vi "ADC Offset Gain_original.vi"(8 "error in (no error)":errorcluster, 9 "Sequence parameters":string[][](array[string])=[["Min limit", "Max limit", "Register sheet file", "Register Sheet"], ["", "", "CC2600.xls", "TX_BLE;Trim"], ["Reg write (addr;value)", "Operating frequency [Hz]", "", ""], ["NA", "2.44G", "", ""]], 10 "Run type":i32, 11 "Method parameters":T3={"Dev"={"Do not disturb DUT"=FALSE, "XOSC"=32000000.0, "Board type"="", "EM"="", "Configure tempboard"=TRUE, "Device specific info"=[], "Generic Object"=refnum}, "Method"={"Run type"=1, "Test name"="Current LPM2 4", "Comment"="", "Results folder"="", "AFC"=enum."Off", "Method name"="Current LPM2 4", "Method results"={"Excel brief report"=FALSE, "Spotfire report"=FALSE, "Starfish report"=FALSE}, "Operator"="", "Reference time"=timestamp(0 s since 1904-01-01), "AFC delay"=0.0, "Initialization"=enum."Enabled", "MD5 Sum"="", "HW addon board"=enum."None", "AFC Regsheet"="", "AFC Regfile"=path "", "dummy"=0.0}, "Inst"={"Instr"={"PS1"={"Name"="", "GPIB address"="", "VISA session"=""}, "PS2"={"Name"="", "GPIB address"="", "VISA session"=""}, "TC1"={"Name"="", "GPIB address"="", "VISA session"=""}, "TC2"={"Name"="", "GPIB address"="", "VISA session"=""}, "SA1"={"Name"="", "GPIB address"="", "VISA session"=""}, "SA2"={"Name"="", "GPIB address"="", "VISA session"=""}, "SG1"={"Name"="", "GPIB address"="", "VISA session"=""}, "SG2"={"Name"="", "GPIB address"="", "VISA session"=""}, "SG3"={"Name"="", "GPIB address"="", "VISA session"=""}, "MI1"={"Name"="", "GPIB address"="", "VISA session"=""}, "MI2"={"Name"="", "GPIB address"="", "VISA session"=""}, "SW SA"={"Name"="", "Controller addr"=""}, "SW SG"={"Name"="", "Controller addr"=""}, "MI3"={"Name"="", "GPIB address"="", "VISA session"=""}}, "Switchbox"={"RF Path"=0, "Cal compensation"=enum."TX", "Switchbox gain mode"="", "State"=enum."TX"}, "Instr to control (i.e. SA1)"="Default", "Intrument info string"=""}, "Sequence parameters"=[["Weight", "Min Limit", "Max Limit", "Register Sheet", "", "", "", "", "", "", "", "", ""], ["Vital", "", "1", "LPM2", "", "", "", "", "", "", "", "", ""], ["Resolution", "Reg write (addr;value)", "Chip mode", "Range", "", "", "", "", "", "", "", "", ""], ["u", "NA", "", "auto", "", "", "", "", "", "", "", "", ""]], "Cond"={"Temp logged"=25.0, "VDD1_PS1_6V"=-999.0, "VDD2_PS1_25V"=-999.0, "VDD4_PS2_25V"=-999.0, "VDD3_PS2_6V"=-999.0}, "Meas config"={"X-axis inner loop index"=32000000, "Y-axis outer loop index"=32000000, "X-axis"=[], "Y-axis"=[], "X-axis array req size"=32000000, "Y-axis array req size"=32000000, "Param description"=[], "Use meas clust for reporting"=FALSE, "Parameter index (page)"=0, "X-axis name"="", "Y-axis name"=""}} {"Cond"."VDD3_PS2_6V" format="%.3f"; "Cond"."VDD4_PS2_25V" format="%.3f"; "Cond"."VDD2_PS1_25V" format="%.3f"; "Cond"."VDD1_PS1_6V" format="%.3f"; "Method"."dummy" format="%.1p"; "Method"."AFC delay" format="%.1p"; "Dev"."XOSC" format="%.3p"}) -> (0 "error out":errorcluster, 1 "End method error":T2, 2 "Short Results":string[](array[string])=["0.00", "0.00", "0.00", "0.00"], 3 "Result summary":string[][](array[string])=[["Critical", "Output Power@2405 MHz", "-3", "4", "dBm"], ["Critical", "Output Power@2410 MHz", "-3", "4", "dBm"]])   [LabVIEW 2019]
doc: "[AutoDocStart]Performs crystal accuracy measurements. Measures the offset from ideal frequency. Primarily used for tuning XOSC capacitors and verifying XOSC trims.\n\nSweeping parameters: operating frequency, OSC override value and VDDR level\n\nResults: Offset frequency in ppm[AutoDocEnd]"
uses:
  User Lib/Utilities/Cluster definitions/Method input.ctl
  User Lib/Utilities/Cluster definitions/Device specific info.ctl
  User Lib/Utilities/Controls/Automatic Frequency Compensation types.ctl
  User Lib/Utilities/Controls/Method Reports.ctl
  User Lib/Utilities/Cluster definitions/Method Initialization.ctl
  User Lib/Utilities/Controls/HW addon boards.ctl
  User Lib/Utilities/Cluster definitions/Instr clust.ctl
  User Lib/Utilities/Switchbox control/SwitchBox_State._ENUMctl.ctl
  User Lib/Utilities/Cluster definitions/End method error cluster.ctl
  User Lib/Utilities/Cluster definitions/DUT vdd control.ctl
  User Lib/Utilities/Cluster definitions/DUT VDD4.ctl
  User Lib/Utilities/Cluster definitions/DUT VDD3.ctl
  User Lib/Utilities/Cluster definitions/DUT VDD2.ctl
  User Lib/Utilities/Cluster definitions/DUT VDD1.ctl
  User Lib/Generic chip methods/Classes/Generic_EM/Chameleon/Loki/Loki.lvclass
  5dbb33b4-abf2-4dec-afba-afc32014483e.vi
  7ebe6cd1-31d9-46d5-9500-a426c9f4248b.vi
  <vilib>/Utility/error.llb/Clear Errors.vi
  User Lib/Generic chip methods/Classes/Generic_EM/Chameleon/65nm.lvclass
  C:/Kharon/User Lib/Generic chip methods/Classes/Generic_EM/Generic_EM/Generic_EM.lvclass
  User Lib/Generic chip methods/board_to_chip_type.vi
  User Lib/Generic chip methods/Classes/Get_Class_init.vi
  User Lib/Generic chip methods/Classes/Generic_EM/Generic_EM/Generic_EM.lvclass
  <vilib>/Analysis/NI_AALPro.lvlib
panel:
  out "Max":u32
  out "Min":u32
  in  "Tab Control":T1(tab)
  out "Output Response [All DUTs]":u32[][](array[numeric])
  out "Measure Codes":dbl[](array[numeric])
  out "intercept":dbl
  out "slope":dbl
  out "Offset Error (mV)":dbl
  out "Gain Error (LSB)":dbl
  # "°C"
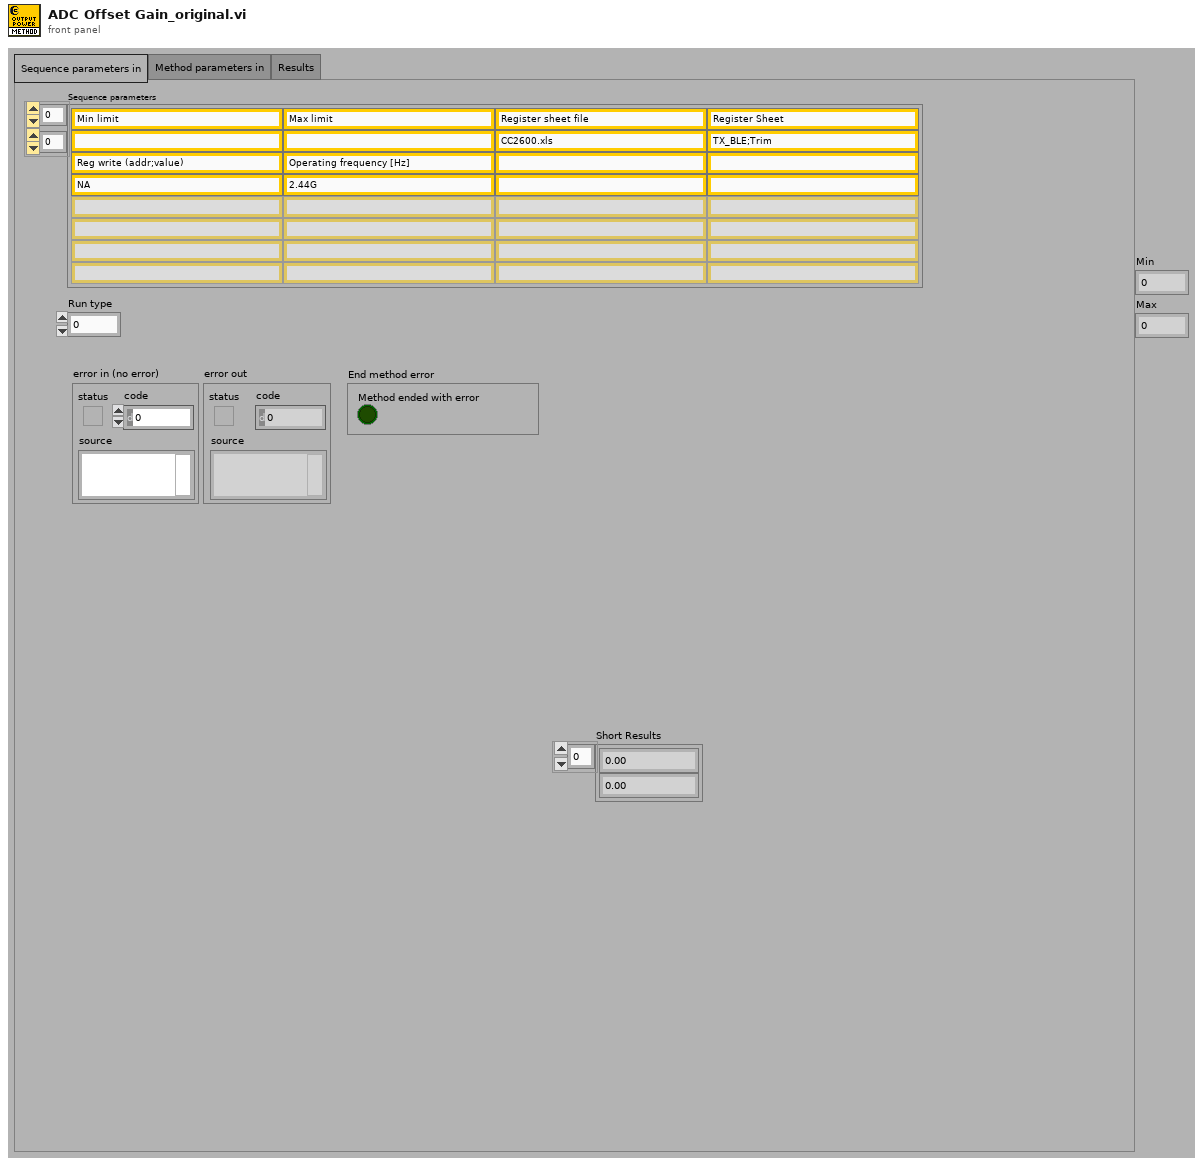
[diagram p1: front panel]
types:
  T1 = enum32{"Sequence parameters in", "Method parameters in", "Results"}
  T2 = typedef "End method error cluster.ctl" = cluster{"Method ended with error":bool}
  T3 = typedef "Method input.ctl" = cluster{"Dev":cluster{"Do not disturb DUT":bool, "XOSC":dbl, "Board type":string, "EM":string, "Configure tempboard":bool, "Device specific info":T4[], "Generic Object":refnum<class>}, "Method":cluster{"Run type":i32, "Test name":string, "Comment":string, "Results folder":string, "AFC":T5, "Method name":string, "Method results":T6, "Operator":string, "Reference time":timestamp, "AFC delay":dbl, "Initialization":T7, "MD5 Sum":string, "HW addon board":T8, "AFC Regsheet":string, "AFC Regfile":path, "dummy":dbl}, "Inst":T9, "Sequence parameters":string[][], "Cond":cluster{"Temp logged":dbl, "VDD1_PS1_6V":dbl, "VDD2_PS1_25V":dbl, "VDD4_PS2_25V":dbl, "VDD3_PS2_6V":dbl}, "Meas config":cluster{"X-axis inner loop index":i32, "Y-axis outer loop index":i32, "X-axis":string[], "Y-axis":string[], "X-axis array req size":i32, "Y-axis array req size":i32, "Param description":string[][], "Use meas clust for reporting":bool, "Parameter index (page)":i32, "X-axis name":string, "Y-axis name":string}}
  T4 = typedef "Device specific info.ctl" = cluster{"EM number":u8, "IP address":string, "Enabled":bool, "Slot no":u8, "RF path":u8, "EM name":string, "Wafer info":string, "AFC frequency ppm":dbl, "Register writes":string[][], "Meas data":string[][][], "Device comment":string}
  T5 = typedef "Automatic Frequency Compensation types.ctl" = enum16{"Off", "Compensate Instrument frequency", "Compensate DUT frequency", "Predictive - Compensate Instrument frequency", "Predictive - Compensate DUT frequency", "Do not skip re-init - Compensate Instrument frequency", "Do not skip re-init - Compensate DUT frequency"}
  T6 = typedef "Method Reports.ctl" = cluster{"Excel brief report":bool, "Spotfire report":bool, "Starfish report":bool}
  T7 = typedef "Method Initialization.ctl" = enum16{"Enabled", "Skip Instr and Device Init", "Enabled with Separate Flash", "Set PS, Device Init and Skip Instr Init", "Skip Device Init"}
  T8 = typedef "HW addon boards.ctl" = enum16{"None", "Current meas 5EM", "Stresstest 10EM"}
  T9 = typedef "Instr clust.ctl" = cluster{"Instr":cluster{"PS1":cluster{"Name":string, "GPIB address":string, "VISA session":refnum<visa-resource-name>}, "PS2":cluster{"Name":string, "GPIB address":string, "VISA session":refnum<visa-resource-name>}, "TC1":cluster{"Name":string, "GPIB address":string, "VISA session":refnum<visa-resource-name>}, "TC2":cluster{"Name":string, "GPIB address":string, "VISA session":refnum<visa-resource-name>}, "SA1":cluster{"Name":string, "GPIB address":string, "VISA session":refnum<visa-resource-name>}, "SA2":cluster{"Name":string, "GPIB address":string, "VISA session":refnum<visa-resource-name>}, "SG1":cluster{"Name":string, "GPIB address":string, "VISA session":refnum<visa-resource-name>}, "SG2":cluster{"Name":string, "GPIB address":string, "VISA session":refnum<visa-resource-name>}, "SG3":cluster{"Name":string, "GPIB address":string, "VISA session":refnum<visa-resource-name>}, "MI1":cluster{"Name":string, "GPIB address":string, "VISA session":refnum<visa-resource-name>}, "MI2":cluster{"Name":string, "GPIB address":string, "VISA session":refnum<visa-resource-name>}, "SW SA":cluster{"Name":string, "Controller addr":string}, "SW SG":cluster{"Name":string, "Controller addr":string}, "MI3":cluster{"Name":string, "GPIB address":string, "VISA session":refnum<visa-resource-name>}}, "Switchbox":cluster{"RF Path":i32, "Cal compensation":enum16{"TX", "RX", "Interferer", "No compensation", "Interferer2"}, "Switchbox gain mode":string, "State":T10}, "Instr to control (i.e. SA1)":string, "Intrument info string":string}
  T10 = typedef "SwitchBox_State._ENUMctl.ctl" = enum16{"TX", "RX", "SP:TX", "SP:RX", "SW:TX", "SW:RX"}
  T11 = typedef "DUT vdd control.ctl" = cluster{"VDD4 config":T12, "VDD3 config":T13, "VDD2 config":T14, "VDD1 config":T15}
  T12 = typedef "DUT VDD4.ctl" = u16
  T13 = typedef "DUT VDD3.ctl" = u16
  T14 = typedef "DUT VDD2.ctl" = u16
  T15 = typedef "DUT VDD1.ctl" = u16
  T16 = typedef "TFW ResponseData.ctl" = cluster{"errorCode":u32, "executionTime":u32, "processedCmdWord":u32, "responsePar":u32[], "actionCode":u32, "cmdStatus":u16}
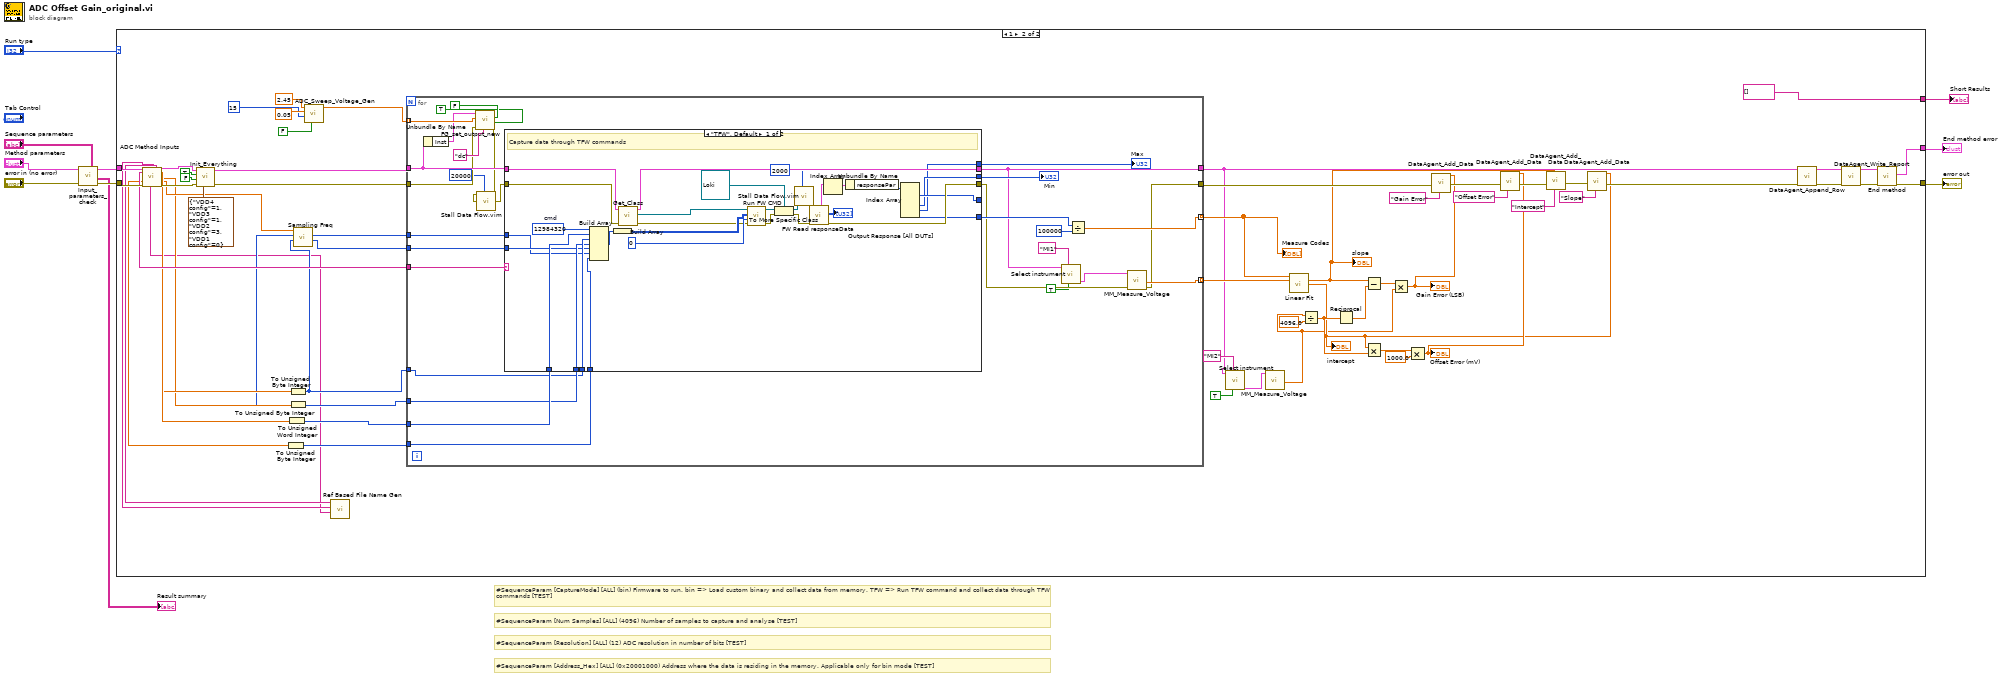
[diagram p0: block diagram]
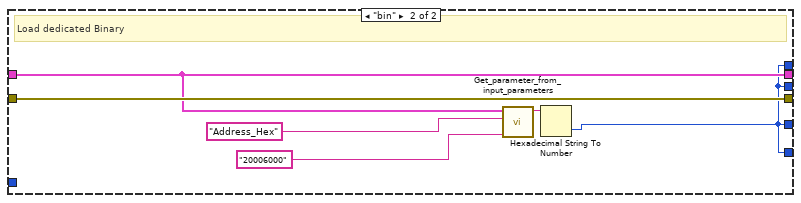
[diagram p3: hidden frame]
diagram:
  # "#SequenceParam [Num Samples] [ALL] (4096) Number of samples to capture and analyse [TEST]"
  # "#SequenceParam [CaptureMode] [ALL] (bin) Firmware to run. bin => Load custom binary and collect data from memory. TFW => Run TFW command and collect data through TFW commands [TEST]"
  # "#SequenceParam [Address_Hex] [ALL] (0x20001000) Address where the data is residing in the memory. Applicable only for bin mode [TEST]"
  # "#SequenceParam [Resolution] [ALL] (12) ADC resolution in number of bits [TEST]"
  n1 = call "Input_parameters_check.vi"("Sequence parameters"="Sequence parameters", "error in"="error in (no error)", "Method cluster in"="Method parameters") -> ("error out"=w9:errorcluster, "Result summary"=→"Result summary":string[][], "Method cluster out"=w5:T3)  [unwired: 6 in]
  n2 = case shown="1" "Run type" {
    tunnel: w9 -> [w11 w59]
    tunnel: [w11 w73] -> w10
    tunnel: w5 -> [_ w60]
    tunnel: [_ w72] -> w4
    tunnel: [_ string[] []] -> w1
    frame 0, Default {
      # "Run type 0 is only for formatting the result summary"
    }
    frame 1 {
      n3 = call "ADC Method Inputs.vi"("Method cluster in"=w60, "error in (no error)"=w59) -> ("Capture Mode"=w56:string, "ADC Channel No."=w47:dbl, "Sampling Freq String"=w43:string, "Resolution String"=w44:string, "Voltage Ref String"=w45:string, "Method cluster out"=w57:T3, "Num Samples"=w55:dbl, "Resolution"=w54:dbl, "Voltage Ref"=w52:dbl, "Sampling Freq"=w53:dbl, "error out"=w58:errorcluster)  [unwired: 6 in, 1 out]
      n4 = call "Init_Everything.vi"("VDD config"=T11 {"VDD4 config"=1, "VDD3 config"=1, "VDD2 config"=3, "VDD1 config"=0}, "error in"=w58, "Support current measurement?"=FALSE, "Override VDD Config"=TRUE, "Method cluster In"=w57) -> ("error out"=w68:errorcluster, "Method cluster out"=w67:T3)  [unwired: 3 in, 2 out]
      n5 = To Unsigned Byte Integer(number=w47) -> (unsigned 8bit integer=w48:u8)
      n6 = To Unsigned Word Integer(number=w55) -> (unsigned 16bit integer=w65:u16)
      n7 = To Unsigned Byte Integer(number=w54) -> (unsigned 8bit integer=w46:u8)
      n8 = To Unsigned Byte Integer(number=w52) -> (unsigned 8bit integer=w49:u8)
      n9 = call "Sampling Freq.vi"("Resolution"=w46, "Voltage Ref"=w49, "Sampling Freq"=w53) -> ("LGPT Count"=w51:u16, "SCOMP"=w50:u16)  [unwired: 7 in]
      n10 = call "ADC_Sweep_Voltage_Gen.vi"("Shuffle"=FALSE, "Count"=15, "Vn"=0.05, "Vp"=2.45) -> ("Vin_Array_Set"=w32:dbl[])  [unwired: 7 in]
      n11 = call "Ref Based File Name Gen.vi"("Sampling Freq String"=w43, "Resolution String"=w44, "Voltage Ref String"=w45) -> ()  [unwired: 8 in, 1 out]
      n12 = for {
        tunnel: w65 -> [w102]
        tunnel: w56 -> [w101]
        tunnel: w51 -> [w100]
        tunnel: w50 -> [w99]
        tunnel: w49 -> [w98]
        tunnel: w48 -> [w97]
        tunnel: w46 -> [w96]
        tunnel: w67 -> [w95]
        tunnel: [w75] -> w13
        tunnel: w68 -> [w91]
        tunnel: [w78] -> w39
        tunnel: w32 -> [w90] mode=indexing
        tunnel: [w88] -> w25 mode=indexing
        tunnel: [w80] -> w17 mode=indexing
        n13 = Unbundle By Name(w95) -> ("Inst"=w89:T9)
        n14 = call "FG_set_output_new.vi"("High impedance (T)"=TRUE, "Invert output"=FALSE, "Function (DC, Sine, Square, Triangle, Ramp up, Ramp down, Pulse)"="dc", "error in"=w91, "High voltage (or DC)"=w90, "InstrCluster in"=w89) -> ("error out"=w82:errorcluster)  [unwired: 4 in, 1 out]
        n15 = call "Stall Data Flow.vim"("value in"=w82, "milliseconds to wait"=u32 20000) -> ("value out"=w83:errorcluster)  [unwired: 1 out]
        n16 = case shown="\"TFW\", Default" w101 {
          tunnel: [w133 w135] -> w75
          tunnel: [w126 w139] -> w79
          tunnel: w83 -> [w125 w139]
          tunnel: w95 -> [w132 w135]
          tunnel: [w114 w134] -> _
          tunnel: w102 -> [w129 _]
          tunnel: w96 -> [w113 _]
          tunnel: w98 -> [w112 _]
          tunnel: w100 -> [w111 _]
          tunnel: w99 -> [w110 _]
          tunnel: w97 -> [w109 _]
          tunnel: [w108 w134] -> w87
          tunnel: [w107 w134] -> w85
          tunnel: [w106 w134] -> w84
          frame "TFW", Default {
            w130 = u32 12984320  # cmd
            # "Capture data through TFW commands"
            n17 = Build Array(w130, w129, w113, w112, w111, w110, w109) -> (w128:u32[])
            n18 = Build Array(w128) -> (w127:u32[][])
            n19 = call "Get_Class.vi"("error in (no error)"=w125, "Method cluster in"=w132) -> ("error out"=w123:errorcluster, "Class Out"=w122:refnum<class "Generic_EM.lvclass">, "Method cluster out"=w133:T3)  [unwired: 6 in, 1 out]
            n20 = call-dynamic "Run FW CMD.vi"("error in (no error)"=w123, "Handler"=u8 0, "cmdBuf"=w127, "Generic_EM in"=w122) -> ("error out"=w119:errorcluster, "Generic_EM out"=w121:refnum<class "Generic_EM.lvclass">)  [unwired: 6 in]
            n21 = To More Specific Class(target class=refnum<class "Loki.lvclass"> refnum ("Loki in"), reference=w121, error in=w119) -> (specific class reference=w105:refnum<class "Loki.lvclass">, error out=w118:errorcluster)
            n22 = call "Stall Data Flow.vim"("value in"=w105, "milliseconds to wait"=u32 2000) -> ("value out"=w104:refnum<class "Loki.lvclass">)  [unwired: 1 out]
            n23 = call "FW Read responseData.vi"("error in (no error)"=w118, "Loki in"=w104) -> ("error out"=w126:errorcluster, "Output Response [All DUTs]"=→"Output Response [All DUTs]":u32[][], "Response"=w116:T16[])  [unwired: 6 in, 1 out]
            n24 = Index Array(array=w116) -> (element=w117:T16)  [unwired: 1 in]
            n25 = Unbundle By Name(w117) -> ("responsePar"=w115:u32[])
            n26 = Index Array(array=w115) -> (element #1=w114:u32, element #3=w107:u32, element #4=w106:u32, element #5=w108:u32)  [unwired: 5 in, 1 out]
          }
          frame "bin" {
            # "Load dedicated Binary"
            n27 = call "Get_parameter_from_input_parameters.vi"("Default value (used if not specified on Front Panel)"="20006000", "Parameter name"="Address_Hex" ("SA_ param name"), "Method cluster (if input param empty)"=w135) -> ("value as String"=w138:string)  [unwired: 2 in, 6 out]
            n28 = Hexadecimal String To Number(string=w138) -> (number=w134:u32)  [unwired: 2 in, 1 out]
          }
        }
        "Min" <- w85
        "Max" <- w84
        n29 = call "Select instrument.vi"("Method cluster (T) / Instr cluster (F)"=TRUE, "Instr.Instr to control (i.e. SA1)"="MI1", "Method cluster in"=w75) -> ("Instr out"=w77:T9)  [unwired: 6 in, 2 out]
        n30 = Divide(x=w87, y=u32 100000) -> (x/y=w88:dbl)
        n31 = call "MM_Measure_Voltage.vi"("error in"=w79, "InstrCluster in"=w77) -> ("error out"=w78:errorcluster, "Measured value"=w80:dbl)  [unwired: 5 in, 3 out]
      }
      "Measure Codes" <- w25
      n32 = call "Select instrument.vi"("Method cluster (T) / Instr cluster (F)"=TRUE, "Instr.Instr to control (i.e. SA1)"="MI2", "Method cluster in"=w13) -> ("Instr out"=w15:T9)  [unwired: 6 in, 2 out]
      n33 = call "MM_Measure_Voltage.vi"("InstrCluster in"=w15) -> ("Measured value"=w14:dbl)  [unwired: 6 in, 4 out]
      n34 = call <vilib>:"Linear Fit.vi"("Y"=w25, "X"=w17) -> ("slope"=w19:dbl, "intercept"=w18:dbl)  [unwired: 9 in, 3 out]
      "intercept" <- w18
      "slope" <- w19
      n35 = Divide(x=w14, y=4096.0) -> (x/y=w27:dbl)
      n36 = Reciprocal(x=w27) -> (1/x=w26:dbl)
      n37 = Subtract(x=w19, y=w26) -> (x-y=w28:dbl)
      n38 = Multiply(x=w18, y=w27) -> (x*y=w30:dbl)
      n39 = Multiply(x=w28, y=w14) -> (x*y=w24:dbl)
      "Gain Error (LSB)" <- w24
      n40 = Multiply(x=w30, y=1000.0) -> (x*y=w23:dbl)
      "Offset Error (mV)" <- w23
      n41 = call "DataAgent_Add_Data.vi"("ColumnName"="Gain Error", "Data"=w24, "error in (no error)"=w39) -> ("error out"=w40:errorcluster)  [unwired: 8 in]
      n42 = call "DataAgent_Add_Data.vi"("ColumnName"="Offset Error", "Data"=w23, "error in (no error)"=w40) -> ("error out"=w41:errorcluster)  [unwired: 8 in]
      n43 = call "DataAgent_Add_Data.vi"("ColumnName"="Intercept", "Data"=w19, "error in (no error)"=w41) -> ("error out"=w22:errorcluster)  [unwired: 8 in]
      n44 = call "DataAgent_Add_Data.vi"("ColumnName"="Slope", "Data"=w18, "error in (no error)"=w22) -> ("error out"=w21:errorcluster)  [unwired: 8 in]
      n45 = call "DataAgent_Append_Row.vi"("error in (no error)"=w21, "Method cluster in"=w13) -> ("error out"=w63:errorcluster, "Method cluster out"=w64:T3)  [unwired: 8 in]
      n46 = call "DataAgent_Write_Report.vi"("error in (no error)"=w63, "Method cluster in"=w64) -> ("error out"=w70:errorcluster, "Method cluster out"=w69:T3)  [unwired: 8 in]
      n47 = call "End method.vi"("error in"=w70, "Method cluster in"=w69) -> ("error out"=w73:errorcluster, "End method error"=w72:T2)  [unwired: 7 in, 1 out]
    }
  }
  "error out" <- w10
  "End method error" <- w4
  "Short Results" <- w1
